vi "LinearPlntInvFF_GetR_Single.vi"(9 "Row":i32, 11 "Linear Plnt Inversion FF":T1) -> (3 "R":dbl)   [LabVIEW 2019, in "Trajectory_Library.lvlib"]
doc: "Returns an element of the current reference vector r.\n \nInputs:\n - LinearPlntInversionFF -- system data cluster\n - row -- Row of r.\n\nOutputs:\n - R -- The row of the current reference vector."
uses:
  Trajectory_Library.lvlib
  LINEAR_PLANT_INV_FF.ctl
  <vilib>/Analysis/Matrix/Datatypes/RealMatrix.ctl
  <vilib>/Analysis/Matrix/NI_Matrix.lvlib
panel:
  # "<States,1>"
  # "<Inputs,1>"
  # "<States,Inputs>"
  # "<States,States>"
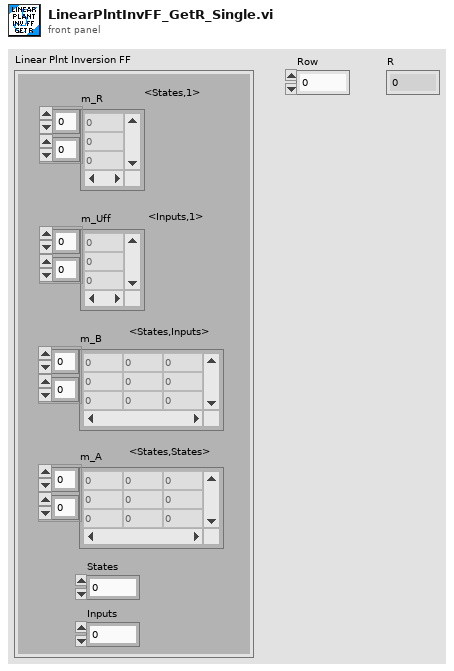
[diagram p1: front panel]
types:
  T1 = typedef "Trajectory_Library.lvlib/LINEAR_PLANT_INV_FF.ctl" = cluster{"m_R":T2, "m_Uff":T2, "m_B":T2, "m_A":T2, "States":i32, "Inputs":i32}
  T2 = typedef "NI_Matrix.lvlib/RealMatrix.ctl" = dbl[][]
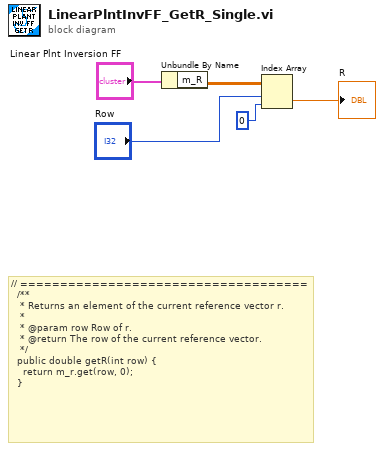
[diagram p0: block diagram]
diagram:
  # "// ====================================\n  /**\n   * Returns an element of the current reference vector r.\n   *\n   * @param row Row of r.\n   * @return The row of the current reference vector.\n   */\n  public double getR(int row) {\n    return m_r.get(row, 0);\n  }"
  n1 = Unbundle By Name("Linear Plnt Inversion FF") -> ("m_R"=w4:T2)
  n2 = Index Array(array=w4, index (row)="Row", index (col)=0) -> (element=→"R":dbl)
